vi "RunningSpeedReward_RotaryEncoder_AP.vi"() -> ()   [LabVIEW 2013]
uses:
  <vilib>/DAQmx/read.llb/DAQmx Read.vi
  <vilib>/DAQmx/read.llb/DAQmx Read (Analog 1D Wfm NChan NSamp).vi
  <vilib>/DAQmx/write.llb/DAQmx Write (Analog 1D DBL 1Chan NSamp).vi
  <vilib>/DAQmx/write.llb/DAQmx Write (Analog DBL 1Chan 1Samp).vi
  <vilib>/DAQmx/create/channels.llb/DAQmx Create Channel (AO-Voltage-Basic).vi
  <vilib>/DAQmx/configure/timing.llb/DAQmx Timing (Sample Clock).vi
  <vilib>/DAQmx/create/channels.llb/DAQmx Create Channel (AI-Voltage-Basic).vi
  <vilib>/DAQmx/miscellaneous.llb/DAQmx Fill In Error Info.vi
  <resource>/objmgr/daqmx.rc
panel:
  out "elapsed time":dbl
  out "start time":timestamp
  out "lick":waveform(dbl)(graph)
  out "reward":waveform(dbl)(graph)
  out "speed":waveform(dbl)(graph)
  in  "encoder ctr0 on:":tag="Dev5"
  out "Raw Speed":dbl[](graph)
  out "distince til reward":dbl
  in  "Manual Reward":bool
  in  "Read Inputs":tag="Dev5/ai0:2"
  in  "Distance?":bool
  out "Speed (cm/s)":dbl
  in  "stop":bool
  in  "Distance (cm)":dbl=50.0
  out "Distance (cm)":dbl
  in  "Reward Output":tag="Dev5/ao1"
  out "reward time":u32
  in  "Speed Output":tag="Dev5/ao0"
  out "new pos":dbl
  out "old pos":dbl
  out "new time":u32
  out "old time":u32
  in  "Interval (s)":dbl=1.0
  in  "Speed (cm/s)":dbl=40.0
  # "DAQ Channels"
  # "Reward Parameters"
  # "Troubleshooting"
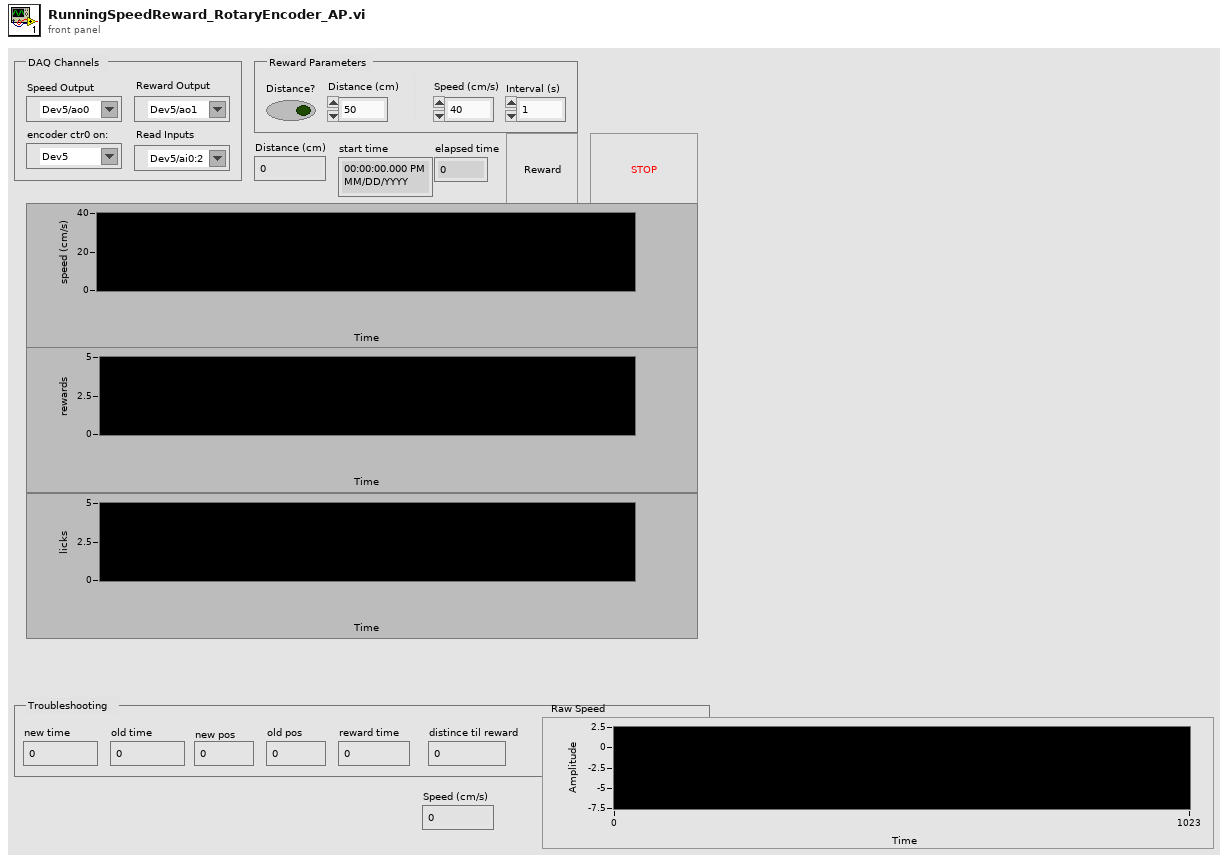
[diagram p1: front panel]
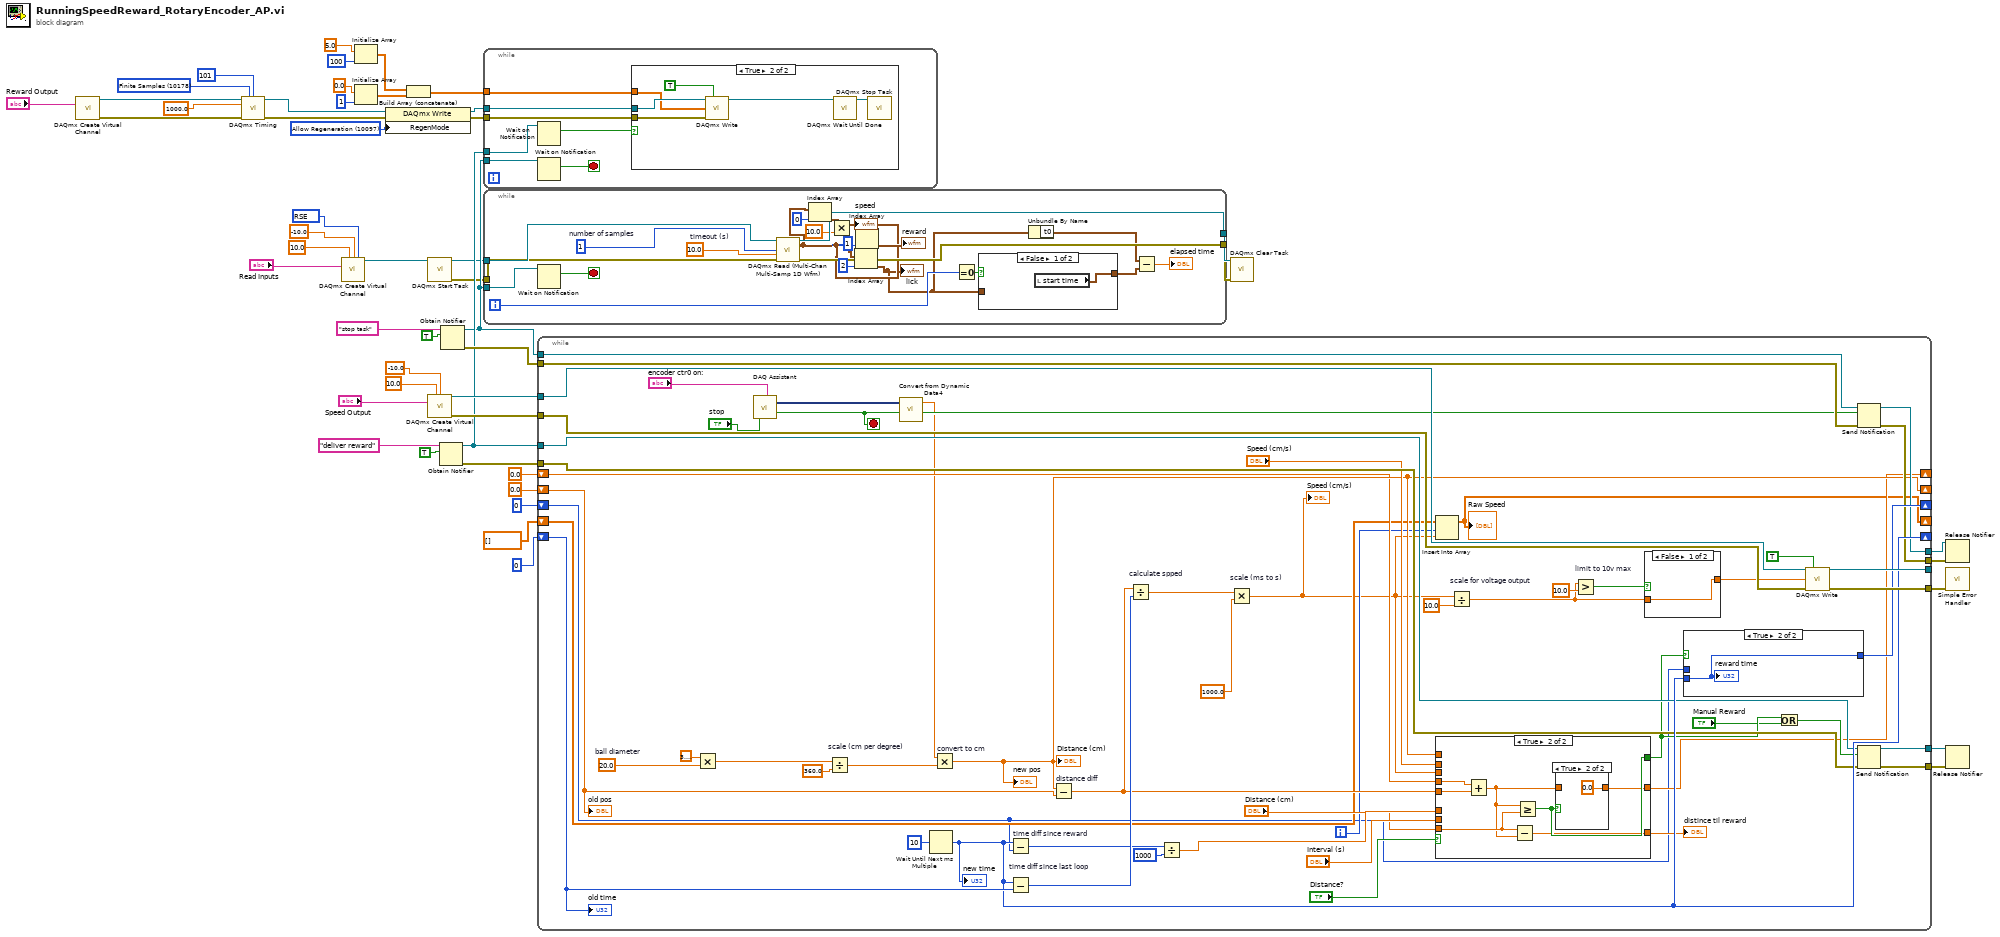
[diagram p0: block diagram]
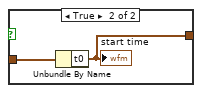
[diagram p2: hidden frame]
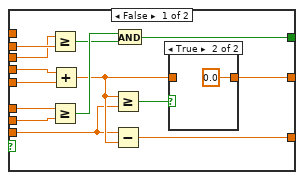
[diagram p4: hidden frame]
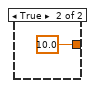
[diagram p7: hidden frame]
diagram:
  w12 = 10083 items=["default"=-1, "RSE"=10083, "NRSE"=10078, "Differential"=10106, "Pseudodifferential"=12529] ("input terminal configuration")
  w25 = 10178 items=["Finite Samples"=10178, "Continuous Samples"=10123, "Hardware Timed Single Point"=12522] ("sample mode")
  w27 = 10097 items=["Allow Regeneration"=10097, "Do Not Allow Regeneration"=10158] ("RegenMode")
  n1 = call-poly <vilib>:"DAQmx Create Virtual Channel.vi"("physical channels"="Reward Output") -> ("task out"=w23:refnum<k21>, "error out"=w21:errorcluster)  [unwired: 13 in]
  n2 = call-poly <vilib>:"DAQmx Timing.vi"("task/channels in"=w23, "sample mode"=w25, "samples per channel"=101, "rate"=1000.0, "error in"=w21) -> ("task out"=w22:refnum<k21>, "error out"=w20:errorcluster)  [unwired: 9 in]
  n3 = call-poly <vilib>:"DAQmx Create Virtual Channel.vi"("maximum value"=10.0 ("Max Voltage"), "minimum value"=-10.0 ("Min Voltage"), "input terminal configuration"=w12, "physical channels"="Read Inputs") -> ("task out"=w8:refnum<k21>)  [unwired: 10 in, 1 out]
  n4 = Initialize Array(5.0 ("element"), 100 ("dimension size")) -> (w29:dbl[])
  n5 = Initialize Array(0.0 ("element"), 1 ("dimension size")) -> (w28:dbl[])
  n6 = property class="DAQmx Write"(reference=w22, error in=w20, "RegenMode"=w27) -> (reference out=w19:refnum<k21>, error out=w18:errorcluster)
  n7 = Build Array (concatenate)(w29, w28) -> (w17:dbl[])
  n8 = call <vilib>:"DAQmx Start Task.vi"("task/channels in"=w8) -> ("task out"=w7:refnum<k21>, "error out"=w6:errorcluster)  [unwired: 13 in]
  n9 = call-poly <vilib>:"DAQmx Create Virtual Channel.vi"("maximum value"=10.0 ("Max Voltage"), "minimum value"=-10.0 ("Min Voltage"), "physical channels"="Speed Output") -> ("task out"=w47:refnum<k21>, "error out"=w46:errorcluster)  [unwired: 11 in]
  n10 = Obtain Notifier(name (unnamed)="deliver reward", notification data type=TRUE) -> (notifier out=w35:refnum<notifier>, error out=w41:errorcluster)  [unwired: 2 in, 1 out]
  n11 = Obtain Notifier(name (unnamed)="stop task", notification data type=TRUE) -> (notifier out=w15:refnum<notifier>, error out=w38:errorcluster)  [unwired: 2 in, 1 out]
  n12 = while {
    tunnel: w35 -> [w57]
    tunnel: w15 -> [w52]
    tunnel: w19 -> [w56]
    tunnel: w18 -> [w55]
    tunnel: w17 -> [w54]
    stop <- w51 stop-if-true
    n13 = Wait on Notification(notifier=w57) -> (notification=w53:bool)  [unwired: 1 in, 5 out]
    n14 = Wait on Notification(notifier=w52) -> (notification=w51:bool)  [unwired: 1 in, 5 out]
    n15 = case shown="True" w53 {
      tunnel: w56 -> [_ w63]
      tunnel: w55 -> [_ w62]
      tunnel: w54 -> [_ w61]
      frame False {
      }
      frame True {
        n16 = call-poly <vilib>:"DAQmx Write.vi"("task/channels in"=w63, "auto start"=TRUE, "data"=w61, "error in"=w62) -> ("task out"=w59:refnum<k21>)  [unwired: 9 in, 2 out]
        n17 = call <vilib>:"DAQmx Wait Until Done.vi"("task/channels in"=w59) -> ("task out"=w58:refnum<k21>)  [unwired: 13 in, 1 out]
        n18 = call <vilib>:"DAQmx Stop Task.vi"("task/channels in"=w58) -> ()  [unwired: 1 in, 14 out]
      }
    }
  }
  n19 = while {
    tunnel: w15 -> [w83]
    tunnel: w7 -> [w79]
    tunnel: [w81] -> w10
    tunnel: [w80] -> w9
    tunnel: w6 -> [w78]
    i -> [w68]
    stop <- w84 stop-if-true
    w82 = 10.0  # timeout (s)
    w85 = 1  # number of samples
    n20 = Wait on Notification(notifier=w83) -> (notification=w84:bool)  [unwired: 1 in, 5 out]
    n21 = call-poly "DAQmx Read (Multi-Chan Multi-Samp 1D Wfm).vi"("task/channels in"=w79, "number of samples per channel"=w85, "timeout"=w82, "error in"=w78) -> ("task out"=w81:refnum<k21>, "data"=w70:waveform(dbl)[], "error out"=w80:errorcluster)  [unwired: 9 in]
    n22 = Index Array(array=w70, index=0) -> (element=w76:waveform(dbl))
    n23 = Multiply(x=w76, y=10.0) -> (x*y=→"speed":waveform(dbl))
    n24 = Index Array(array=w70, index=2) -> (element=w67:waveform(dbl))
    "lick" <- w67
    n25 = Index Array(array=w70, index=1) -> (element=→"reward":waveform(dbl))
    n26 = Equal To 0?(x=w68) -> (x = 0?=w69:bool)
    n27 = case shown="False" w69 {
      tunnel: w67 -> [_ w88]
      tunnel: [w86 w87] -> w65
      frame False {
        n28 = local read "start time"() -> (w86:timestamp)
      }
      frame True {
        n29 = Unbundle By Name(w88) -> ("t0"=w87:timestamp)
        "start time" <- w87
      }
    }
    n30 = Unbundle By Name(w67) -> ("t0"=w66:timestamp)
    n31 = Subtract(x=w66, y=w65) -> (x-y=→"elapsed time":dbl)
  }
  n32 = while {
    shift-right: [w133] -> _
    shift-left: u32 0 ("millisecond timer value") -> [w144]
    shift-right: [w107] -> _
    shift-left: 0.0 -> [w143]
    tunnel: [w137] -> _
    tunnel: [w136] -> w16
    tunnel: w47 -> [w135]
    shift-right: [w129] -> _
    shift-left: u32 0 ("millisecond timer value") -> [w90]
    tunnel: w46 -> [w128]
    tunnel: w35 -> [w120]
    tunnel: w41 -> [w127]
    tunnel: [w126] -> w39
    tunnel: [w125] -> w40
    tunnel: w15 -> [w124]
    tunnel: w38 -> [w123]
    tunnel: [w122] -> w37
    tunnel: [w121] -> w36
    shift-right: [w102] -> _
    shift-left: 0.0 ("y") -> [w101]
    shift-right: [w89] -> _
    shift-left: dbl[] [] -> [w93]
    i -> [w94]
    stop <- w119 stop-if-true
    w99 = 20.0  # ball diameter
    n33 = Multiply(x=3.141592653589793, y=w99) -> (x*y=w100:dbl)
    n34 = call "DAQ Assistant"("stop (F)"="stop", "device name"="encoder ctr0 on:") -> ("data"=w91:dynamicdata, "stopped"=w119:bool)  [unwired: 14 in, 2 out]
    n35 = Divide "scale (cm per degree)"(x=w100, y=360.0) -> (x/y=w117:dbl)
    n36 = call "Convert from Dynamic Data4"("Dynamic Data Type"=w91) -> ("Scalar"=w95:dbl)  [unwired: 3 in]
    n37 = Wait Until Next ms Multiple(millisecond multiple=u32 10 ("milliseconds to wait")) -> (millisecond timer value=w133:u32)
    "new time" <- w133
    n38 = Multiply "convert to cm"(x=w95, y=w117) -> (x*y=w107:dbl)
    "new pos" <- w107
    "Distance (cm)" <- w107
    n39 = Subtract "time diff since reward"(x=w133, y=w90) -> (x-y=w131:u32)
    n40 = Subtract "time diff since last loop"(x=w133, y=w144) -> (x-y=w142:u32)
    n41 = Subtract "distance diff"(x=w107, y=w143) -> (x-y=w103:dbl)
    n42 = Divide "calculate spped"(x=w103, y=w142) -> (x/y=w118:dbl)
    n43 = Divide(x=w131, y=u32 1000) -> (x/y=w132:dbl)
    n44 = Multiply "scale (ms to s)"(x=w118, y=1000.0) -> (x*y=w92:dbl)
    "Speed (cm/s)" <- w92
    n45 = Insert Into Array(array=w93, index=w94, new element=w92) -> (w89:dbl[])
    "Raw Speed" <- w89
    n46 = case shown="True" "Distance?" {
      tunnel: w132 -> [w158 _]
      tunnel: w92 -> [w146 _]
      tunnel: [w155 w166] -> w105
      tunnel: "Speed (cm/s)" -> [w154 _]
      tunnel: "Interval (s)" -> [w153 _]
      tunnel: "Distance (cm)" -> [w148 w164]
      tunnel: w107 -> [_ _]
      tunnel: w103 -> [w145 w161]
      tunnel: [w150 w165] -> w102
      tunnel: w101 -> [w149 w167]
      tunnel: [w147 w162] -> w97
      frame False {
        n47 = Greater Or Equal?(x=w146, y=w154) -> (x >= y?=w156:bool)
        n48 = Greater Or Equal?(x=w158, y=w153) -> (x >= y?=w157:bool)
        n49 = Add(x=w149, y=w145) -> (x+y=w151:dbl)
        n50 = Greater Or Equal?(x=w151, y=w148) -> (x >= y?=w152:bool)
        n51 = Subtract(x=w148, y=w151) -> (x-y=w147:dbl)
        n52 = And(x=w157, y=w156) -> (x .and. y?=w155:bool)
        n53 = case shown="True" w152 {
          tunnel: w151 -> [w159 _]
          tunnel: [w159 0.0 ("y")] -> w150
          frame False {
          }
          frame True {
          }
        }
      }
      frame True {
        n54 = Add(x=w167, y=w161) -> (x+y=w163:dbl)
        n55 = Subtract(x=w164, y=w163) -> (x-y=w162:dbl)
        n56 = Greater Or Equal?(x=w163, y=w164) -> (x >= y?=w166:bool)
        n57 = case shown="True" w166 {
          tunnel: w163 -> [w168 _]
          tunnel: [w168 0.0 ("y")] -> w165
          frame False {
          }
          frame True {
          }
        }
      }
    }
    "distince til reward" <- w97
    n58 = Divide "scale for voltage output"(x=w92, y=10.0) -> (x/y=w114:dbl)
    n59 = Greater? "limit to 10v max"(x=w114, y=10.0) -> (0:w115:bool)
    n60 = case shown="False" w115 {
      tunnel: w114 -> [w170 _]
      tunnel: [w170 10.0 ("y")] -> w113
      frame False {
      }
      frame True {
      }
    }
    n61 = case shown="True" w105 {
      tunnel: w133 -> [_ w173]
      tunnel: [w172 w173] -> w129
      tunnel: w90 -> [w172 _]
      frame False {
      }
      frame True {
        "reward time" <- w173
      }
    }
    n62 = Or(x=w105, y="Manual Reward") -> (x .or. y?=w106:bool)
    n63 = call-poly <vilib>:"DAQmx Write.vi"("task/channels in"=w135, "auto start"=TRUE, "data"=w113, "error in"=w128) -> ("task out"=w137:refnum<k21>, "error out"=w136:errorcluster)  [unwired: 9 in, 1 out]
    n64 = Send Notification(notification=w119, notifier=w124, error in (no error)=w123) -> (notifier out=w122:refnum<notifier>, error out=w121:errorcluster)
    n65 = Send Notification(notification=w106, notifier=w120, error in (no error)=w127) -> (notifier out=w126:refnum<notifier>, error out=w125:errorcluster)
    "old time" <- w144
    "old pos" <- w143
  }
  n66 = call <vilib>:"DAQmx Clear Task.vi"("task in"=w10, "error in"=w9) -> ()  [unwired: 13 in, 1 out]
  n67 = Release Notifier(notifier=w37, error in (no error)=w36) -> ()  [unwired: 1 in, 3 out]
  n68 = call <vilib>:"Simple Error Handler.vi"("error in (no error)"=w16) -> ()  [unwired: 4 in, 5 out]
  n69 = Release Notifier(notifier=w39, error in (no error)=w40) -> ()  [unwired: 1 in, 3 out]
